vi "Update Leds.vi"(8 "error in (no error)":errorcluster, 11 "GripsMaster in":refnum<class "GripsMaster.lvclass">) -> (0 "error out":errorcluster, 3 "GripsMaster out":refnum<class "GripsMaster.lvclass">)   [LabVIEW 2013, in "GripsMaster.lvclass"]
uses:
  GripsMaster.lvclass
  GripsMaster.lvclass/GripsMaster.ctl
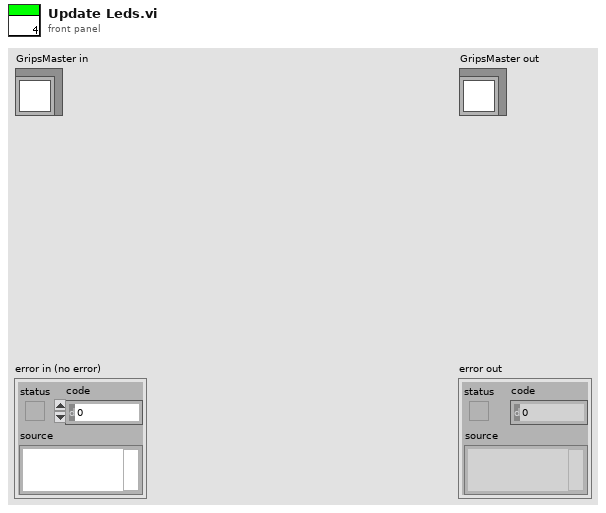
[diagram p1: front panel]
types:
  T1 = typedef "Digital Values.ctl" = cluster{"names":string[], "values":bool[]}
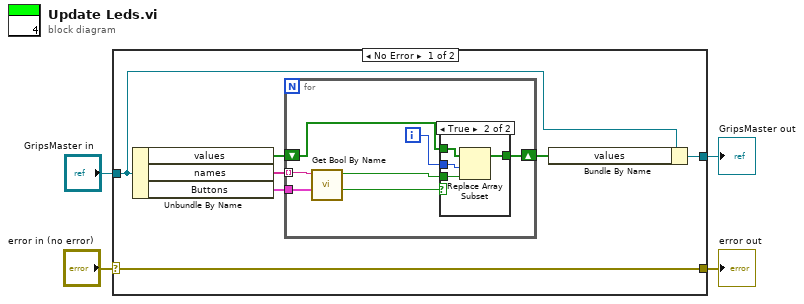
[diagram p0: block diagram]
diagram:
  n1 = case shown="No Error" "error in (no error)" {
    selector: "error in (no error)" -> [w11 w25]
    tunnel: [w11 w25] -> w3
    tunnel: [w7 w24] -> w1
    tunnel: "GripsMaster in" -> [w6 w24]
    frame No Error {
      n2 = Unbundle By Name(w6) -> ("values"=w8:bool[], "names"=w9:string[], "Buttons"=w10:T1)
      n3 = for {
        tunnel: w9 -> [w18] mode=indexing
        shift-right: [w13] -> w5
        shift-left: w8 -> [w15]
        tunnel: w10 -> [w12]
        i -> [w14]
        n4 = call "Get Bool By Name.vi"("name"=w18, "Digital Values"=w12) -> ("result"=w16:bool, "found?"=w17:bool)  [unwired: 7 in]
        n5 = case shown="True" w17 {
          tunnel: [w19 w23] -> w13
          tunnel: w16 -> [_ w20]
          tunnel: w14 -> [_ w22]
          tunnel: w15 -> [w19 w21]
          frame False {
          }
          frame True {
            n6 = Replace Array Subset(array=w21, new element=w20, index=w22) -> (w23:bool[])
          }
        }
      }
      n7 = Bundle By Name(cluster=w6, "values"=w5) -> (w7:refnum<class "GripsMaster.lvclass">)
    }
    frame Error {
    }
  }
  "error out" <- w3
  "GripsMaster out" <- w1
